vi "XMLExtractSheets.vi"(8 "error in (no error)":errorcluster, 11 "byte stream":string="<?xml version=\"1.0\" encoding=\"UTF-8\"?>\n<office:document-content xmlns:office=\"urn:oasis:names:tc:opendocument:xmlns:office:1.0\" xmlns:style=\"urn:oasis:names:tc:opendocument:xmlns:style:1.0\" xmlns:text=\"urn:oasis:names:tc:opendocument:xmlns:text:1.0\" xmlns:table=\"urn:oasis:names:tc:opendocument:xmlns:table:1.0\" xmlns:draw=\"urn:oasis:names:tc:opendocument:xmlns:drawing:1.0\" xmlns:fo=\"urn:oasis:names:tc:opendocument:xmlns:xsl-fo-compatible:1.0\" xmlns:xlink=\"http://www.w3.org/1999/xlink\" xmlns:dc=\"http://purl.org/dc/elements/1.1/\" xmlns:meta=\"urn:oasis:names:tc:opendocument:xmlns:meta:1.0\" xmlns:number=\"urn:oasis:names:tc:opendocument:xmlns:datastyle:1.0\" xmlns:presentation=\"urn:oasis:names:tc:opendocument:xmlns:presentation:1.0\" xmlns:svg=\"urn:oasis:names:tc:opendocument:xmlns:svg-compatible:1.0\" xmlns:chart=\"urn:oasis:names:tc:opendocument:xmlns:chart:1.0\" xmlns:dr3d=\"urn:oasis:names:tc:opendocument:xmlns:dr3d:1.0\" xmlns:math=\"http://www.w3.org/1998/Math/MathML\" xmlns:form=\"urn:oasis:names:tc:opendocument:xmlns:form:1.0\" xmlns:script=\"urn:oasis:names:tc:opendocument:xmlns:script:1.0\" xmlns:ooo=\"http://openoffice.org/2004/office\" xmlns:ooow=\"http://openoffice.org/2004/writer\" xmlns:oooc=\"http://openoffice.org/2004/calc\" xmlns:dom=\"http://www.w3.org/2001/xml-events\" xmlns:xforms=\"http://www.w3.org/2002/xforms\" xmlns:xsd=\"http://www.w3.org/2001/XMLSchema\" xmlns:xsi=\"http://www.w3.org/2001/XMLSchema-instance\" xmlns:rpt=\"http://openoffice.org/2005/report\" xmlns:of=\"urn:oasis:names:tc:opendocument:xmlns:of:1.2\" xmlns:xhtml=\"http://www.w3.org/1999/xhtml\" xmlns:grddl=\"http://www.w3.org/2003/g/data-view#\" xmlns:tableooo=\"http://openoffice.org/2009/table\" xmlns:drawooo=\"http://openoffice.org/2010/draw\" xmlns:calcext=\"urn:org:documentfoundation:names:experimental:calc:xmlns:calcext:1.0\" xmlns:loext=\"urn:org:documentfoundation:names:experimental:office:xmlns:loext:1.0\" xmlns:field=\"urn:openoffice:names:experimental:ooo-ms-interop:xmlns:field:1.0\" xmlns:formx=\"urn:openoffice:names:experimental:ooxml-odf-interop:xmlns:form:1.0\" xmlns:css3t=\"http://www.w3.org/TR/css3-text/\" office:version=\"1.2\"><office:scripts/><office:font-face-decls><style:font-face style:name=\"Liberation Sans\" svg:font-family=\"&apos;Liberation Sans&apos;\" style:font-family-generic=\"swiss\" style:font-pitch=\"variable\"/><style:font-face style:name=\"Mangal\" svg:font-family=\"Mangal\" style:font-family-generic=\"system\" style:font-pitch=\"variable\"/><style:font-face style:name=\"Microsoft YaHei\" svg:font-family=\"&apos;Microsoft YaHei&apos;\" style:font-family-generic=\"system\" style:font-pitch=\"variable\"/><style:font-face style:name=\"Segoe UI\" svg:font-family=\"&apos;Segoe UI&apos;\" style:font-family-generic=\"system\" style:font-pitch=\"variable\"/><style:font-face style:name=\"Tahoma\" svg:font-family=\"Tahoma\" style:font-family-generic=\"system\" style:font-pitch=\"variable\"/></office:font-face-decls><office:automatic-styles><style:style style:name=\"co1\" style:family=\"table-column\"><style:table-column-properties fo:break-before=\"auto\" style:column-width=\"22.58mm\"/></style:style><style:style style:name=\"ro1\" style:family=\"table-row\"><style:table-row-properties style:row-height=\"4.52mm\" fo:break-before=\"auto\" style:use-optimal-row-height=\"true\"/></style:style><style:style style:name=\"ta1\" style:family=\"table\" style:master-page-name=\"Default\"><style:table-properties table:display=\"true\" style:writing-mode=\"lr-tb\"/></style:style></office:automatic-styles><office:body><office:spreadsheet><table:table table:name=\"Sheet1\" table:style-name=\"ta1\"><table:table-column table:style-name=\"co1\" table:number-columns-repeated=\"8\" table:default-cell-style-name=\"Default\"/><table:table-row table:style-name=\"ro1\" table:number-rows-repeated=\"3\"><table:table-cell table:number-columns-repeated=\"8\"/></table:table-row><table:table-row table:style-name=\"ro1\"><table:table-cell/><table:table-cell office:value-type=\"string\" calcext:value-type=\"string\"><text:p>b1</text:p></table:table-cell><table:table-cell office:value-type=\"string\" calcext:value-type=\"string\"><text:p>c1</text:p></table:table-cell><table:table-cell table:number-columns-repeated=\"5\"/></table:table-row><table:table-row table:style-name=\"ro1\"><table:table-cell/><table:table-cell office:value-type=\"string\" calcext:value-type=\"string\"><text:p>b2</text:p></table:table-cell><table:table-cell office:value-type=\"string\" calcext:value-type=\"string\"><text:p>c2</text:p></table:table-cell><table:table-cell table:number-columns-repeated=\"5\"/></table:table-row><table:table-row table:style-name=\"ro1\"><table:table-cell/><table:table-cell office:value-type=\"string\" calcext:value-type=\"string\"><text:p>b3</text:p></table:table-cell><table:table-cell office:value-type=\"string\" calcext:value-type=\"string\"><text:p>c3</text:p></table:table-cell><table:table-cell table:number-columns-repeated=\"5\"/></table:table-row><table:table-row table:style-name=\"ro1\"><table:table-cell/><table:table-cell office:value-type=\"string\" calcext:value-type=\"string\"><text:p>b4</text:p></table:table-cell><table:table-cell office:value-type=\"string\" calcext:value-type=\"string\"><text:p>c4</text:p></table:table-cell><table:table-cell table:number-columns-repeated=\"5\"/></table:table-row><table:table-row table:style-name=\"ro1\"><table:table-cell/><table:table-cell office:value-type=\"string\" calcext:value-type=\"string\"><text:p>b5</text:p></table:table-cell><table:table-cell office:value-type=\"string\" calcext:value-type=\"string\"><text:p>c5</text:p></table:table-cell><table:table-cell table:number-columns-repeated=\"5\"/></table:table-row><table:table-row table:style-name=\"ro1\"><table:table-cell/><table:table-cell office:value-type=\"string\" calcext:value-type=\"string\"><text:p>b6</text:p></table:table-cell><table:table-cell office:value-type=\"string\" calcext:value-type=\"string\"><text:p>c6</text:p></table:table-cell><table:table-cell table:number-columns-repeated=\"5\"/></table:table-row><table:table-row table:style-name=\"ro1\"><table:table-cell/><table:table-cell office:value-type=\"string\" calcext:value-type=\"string\"><text:p>b7</text:p></table:table-cell><table:table-cell office:value-type=\"string\" calcext:value-type=\"string\"><text:p>c7</text:p></table:table-cell><table:table-cell table:number-columns-repeated=\"5\"/></table:table-row><table:table-row table:style-name=\"ro1\"><table:table-cell/><table:table-cell office:value-type=\"string\" calcext:value-type=\"string\"><text:p>b8</text:p></table:table-cell><table:table-cell office:value-type=\"string\" calcext:value-type=\"string\"><text:p>c8</text:p></table:table-cell><table:table-cell table:number-columns-repeated=\"5\"/></table:table-row><table:table-row table:style-name=\"ro1\" table:number-rows-repeated=\"2\"><table:table-cell table:number-columns-repeated=\"8\"/></table:table-row><table:table-row table:style-name=\"ro1\"><table:table-cell table:number-columns-repeated=\"3\"/><table:table-cell office:value-type=\"string\" calcext:value-type=\"string\"><text:p>d1</text:p></table:table-cell><table:table-cell office:value-type=\"string\" calcext:value-type=\"string\"><text:p>e1</text:p></table:table-cell><table:table-cell table:number-columns-repeated=\"3\"/></table:table-row><table:table-row table:style-name=\"ro1\"><table:table-cell table:number-columns-repeated=\"3\"/><table:table-cell office:value-type=\"string\" calcext:value-type=\"string\"><text:p>d2</text:p></table:table-cell><table:table-cell office:value-type=\"string\" calcext:value-type=\"string\"><text:p>e2</text:p></table:table-cell><table:table-cell table:number-columns-repeated=\"3\"/></table:table-row><table:table-row table:style-name=\"ro1\"><table:table-cell table:number-columns-repeated=\"3\"/><table:table-cell office:value-type=\"string\" calcext:value-type=\"string\"><text:p>d3</text:p></table:table-cell><table:table-cell office:value-type=\"string\" calcext:value-type=\"string\"><text:p>e3</text:p></table:table-cell><table:table-cell table:number-columns-repeated=\"3\"/></table:table-row><table:table-row table:style-name=\"ro1\"><table:table-cell table:number-columns-repeated=\"3\"/><table:table-cell office:value-type=\"string\" calcext:value-type=\"string\"><text:p>d4</text:p></table:table-cell><table:table-cell office:value-type=\"string\" calcext:value-type=\"string\"><text:p>e4</text:p></table:table-cell><table:table-cell table:number-columns-repeated=\"3\"/></table:table-row><table:table-row table:style-name=\"ro1\"><table:table-cell table:number-columns-repeated=\"3\"/><table:table-cell office:value-type=\"string\" calcext:value-type=\"string\"><text:p>d5</text:p></table:table-cell><table:table-cell office:value-type=\"string\" calcext:value-type=\"string\"><text:p>e5</text:p></table:table-cell><table:table-cell table:number-columns-repeated=\"3\"/></table:table-row><table:table-row table:style-name=\"ro1\" table:number-rows-repeated=\"14\"><table:table-cell table:number-columns-repeated=\"8\"/></table:table-row><table:table-row table:style-name=\"ro1\"><table:table-cell table:number-columns-repeated=\"5\"/><table:table-cell office:value-type=\"string\" calcext:value-type=\"string\"><text:p>f1</text:p></table:table-cell><table:table-cell/><table:table-cell office:value-type=\"string\" calcext:value-type=\"string\"><text:p>h1</text:p></table:table-cell></table:table-row><table:table-row table:style-name=\"ro1\"><table:table-cell table:number-columns-repeated=\"5\"/><table:table-cell office:value-type=\"string\" calcext:value-type=\"string\"><text:p>f2</text:p></table:table-cell><table:table-cell/><table:table-cell office:value-type=\"string\" calcext:value-type=\"string\"><text:p>h2</text:p></table:table-cell></table:table-row><table:table-row table:style-name=\"ro1\"><table:table-cell table:number-columns-repeated=\"5\"/><table:table-cell office:value-type=\"string\" calcext:value-type=\"string\"><text:p>f3</text:p></table:table-cell><table:table-cell/><table:table-cell office:value-type=\"string\" calcext:value-type=\"string\"><text:p>h3</text:p></table:table-cell></table:table-row><table:table-row table:style-name=\"ro1\"><table:table-cell table:number-columns-repeated=\"5\"/><table:table-cell office:value-type=\"string\" calcext:value-type=\"string\"><text:p>f4</text:p></table:table-cell><table:table-cell/><table:table-cell office:value-type=\"string\" calcext:value-type=\"string\"><text:p>h4</text:p></table:table-cell></table:table-row><table:table-row table:style-name=\"ro1\"><table:table-cell table:number-columns-repeated=\"5\"/><table:table-cell office:value-type=\"string\" calcext:value-type=\"string\"><text:p>f5</text:p></table:table-cell><table:table-cell/><table:table-cell office:value-type=\"string\" calcext:value-type=\"string\"><text:p>h5</text:p></table:table-cell></table:table-row><table:table-row table:style-name=\"ro1\"><table:table-cell table:number-columns-repeated=\"5\"/><table:table-cell office:value-type=\"string\" calcext:value-type=\"string\"><text:p>f6</text:p></table:table-cell><table:table-cell/><table:table-cell office:value-type=\"string\" calcext:value-type=\"string\"><text:p>h6</text:p></table:table-cell></table:table-row><table:table-row table:style-name=\"ro1\"><table:table-cell table:number-columns-repeated=\"5\"/><table:table-cell office:value-type=\"string\" calcext:value-type=\"string\"><text:p>f7</text:p></table:table-cell><table:table-cell/><table:table-cell office:value-type=\"string\" calcext:value-type=\"string\"><text:p>h7</text:p></table:table-cell></table:table-row></table:table><table:table table:name=\"Sheet1_2\" table:style-name=\"ta1\"><table:table-column table:style-name=\"co1\" table:number-columns-repeated=\"8\" table:default-cell-style-name=\"Default\"/><table:table-row table:style-name=\"ro1\" table:number-rows-repeated=\"3\"><table:table-cell table:number-columns-repeated=\"8\"/></table:table-row><table:table-row table:style-name=\"ro1\"><table:table-cell/><table:table-cell office:value-type=\"string\" calcext:value-type=\"string\"><text:p>b1</text:p></table:table-cell><table:table-cell office:value-type=\"string\" calcext:value-type=\"string\"><text:p>c1</text:p></table:table-cell><table:table-cell table:number-columns-repeated=\"5\"/></table:table-row><table:table-row table:style-name=\"ro1\"><table:table-cell/><table:table-cell office:value-type=\"string\" calcext:value-type=\"string\"><text:p>b2</text:p></table:table-cell><table:table-cell office:value-type=\"string\" calcext:value-type=\"string\"><text:p>c2</text:p></table:table-cell><table:table-cell table:number-columns-repeated=\"5\"/></table:table-row><table:table-row table:style-name=\"ro1\"><table:table-cell/><table:table-cell office:value-type=\"string\" calcext:value-type=\"string\"><text:p>b3</text:p></table:table-cell><table:table-cell office:value-type=\"string\" calcext:value-type=\"string\"><text:p>c3</text:p></table:table-cell><table:table-cell table:number-columns-repeated=\"5\"/></table:table-row><table:table-row table:style-name=\"ro1\"><table:table-cell/><table:table-cell office:value-type=\"string\" calcext:value-type=\"string\"><text:p>b4</text:p></table:table-cell><table:table-cell office:value-type=\"string\" calcext:value-type=\"string\"><text:p>c4</text:p></table:table-cell><table:table-cell table:number-columns-repeated=\"5\"/></table:table-row><table:table-row table:style-name=\"ro1\"><table:table-cell/><table:table-cell office:value-type=\"string\" calcext:value-type=\"string\"><text:p>b5</text:p></table:table-cell><table:table-cell office:value-type=\"string\" calcext:value-type=\"string\"><text:p>c5</text:p></table:table-cell><table:table-cell table:number-columns-repeated=\"5\"/></table:table-row><table:table-row table:style-name=\"ro1\"><table:table-cell/><table:table-cell office:value-type=\"string\" calcext:value-type=\"string\"><text:p>b6</text:p></table:table-cell><table:table-cell office:value-type=\"string\" calcext:value-type=\"string\"><text:p>c6</text:p></table:table-cell><table:table-cell table:number-columns-repeated=\"5\"/></table:table-row><table:table-row table:style-name=\"ro1\"><table:table-cell/><table:table-cell office:value-type=\"string\" calcext:value-type=\"string\"><text:p>b7</text:p></table:table-cell><table:table-cell office:value-type=\"string\" calcext:value-type=\"string\"><text:p>c7</text:p></table:table-cell><table:table-cell table:number-columns-repeated=\"5\"/></table:table-row><table:table-row table:style-name=\"ro1\"><table:table-cell/><table:table-cell office:value-type=\"string\" calcext:value-type=\"string\"><text:p>b8</text:p></table:table-cell><table:table-cell office:value-type=\"string\" calcext:value-type=\"string\"><text:p>c8</text:p></table:table-cell><table:table-cell table:number-columns-repeated=\"5\"/></table:table-row><table:table-row table:style-name=\"ro1\" table:number-rows-repeated=\"2\"><table:table-cell table:number-columns-repeated=\"8\"/></table:table-row><table:table-row table:style-name=\"ro1\"><table:table-cell table:number-columns-repeated=\"3\"/><table:table-cell office:value-type=\"string\" calcext:value-type=\"string\"><text:p>d1</text:p></table:table-cell><table:table-cell office:value-type=\"string\" calcext:value-type=\"string\"><text:p>e1</text:p></table:table-cell><table:table-cell table:number-columns-repeated=\"3\"/></table:table-row><table:table-row table:style-name=\"ro1\"><table:table-cell table:number-columns-repeated=\"3\"/><table:table-cell office:value-type=\"string\" calcext:value-type=\"string\"><text:p>d2</text:p></table:table-cell><table:table-cell office:value-type=\"string\" calcext:value-type=\"string\"><text:p>e2</text:p></table:table-cell><table:table-cell table:number-columns-repeated=\"3\"/></table:table-row><table:table-row table:style-name=\"ro1\"><table:table-cell table:number-columns-repeated=\"3\"/><table:table-cell office:value-type=\"string\" calcext:value-type=\"string\"><text:p>d3</text:p></table:table-cell><table:table-cell office:value-type=\"string\" calcext:value-type=\"string\"><text:p>e3</text:p></table:table-cell><table:table-cell table:number-columns-repeated=\"3\"/></table:table-row><table:table-row table:style-name=\"ro1\"><table:table-cell table:number-columns-repeated=\"3\"/><table:table-cell office:value-type=\"string\" calcext:value-type=\"string\"><text:p>d4</text:p></table:table-cell><table:table-cell office:value-type=\"string\" calcext:value-type=\"string\"><text:p>e4</text:p></table:table-cell><table:table-cell table:number-columns-repeated=\"3\"/></table:table-row><table:table-row table:style-name=\"ro1\"><table:table-cell table:number-columns-repeated=\"3\"/><table:table-cell office:value-type=\"string\" calcext:value-type=\"string\"><text:p>d5</text:p></table:table-cell><table:table-cell office:value-type=\"string\" calcext:value-type=\"string\"><text:p>e5</text:p></table:table-cell><table:table-cell table:number-columns-repeated=\"3\"/></table:table-row><table:table-row table:style-name=\"ro1\" table:number-rows-repeated=\"14\"><table:table-cell table:number-columns-repeated=\"8\"/></table:table-row><table:table-row table:style-name=\"ro1\"><table:table-cell/><table:table-cell office:value-type=\"string\" calcext:value-type=\"string\"><text:p>f1</text:p></table:table-cell><table:table-cell table:number-columns-repeated=\"5\"/><table:table-cell office:value-type=\"string\" calcext:value-type=\"string\"><text:p>h1</text:p></table:table-cell></table:table-row><table:table-row table:style-name=\"ro1\"><table:table-cell/><table:table-cell office:value-type=\"string\" calcext:value-type=\"string\"><text:p>f2</text:p></table:table-cell><table:table-cell table:number-columns-repeated=\"5\"/><table:table-cell office:value-type=\"string\" calcext:value-type=\"string\"><text:p>h2</text:p></table:table-cell></table:table-row><table:table-row table:style-name=\"ro1\"><table:table-cell/><table:table-cell office:value-type=\"string\" calcext:value-type=\"string\"><text:p>f3</text:p></table:table-cell><table:table-cell table:number-columns-repeated=\"5\"/><table:table-cell office:value-type=\"string\" calcext:value-type=\"string\"><text:p>h3</text:p></table:table-cell></table:table-row><table:table-row table:style-name=\"ro1\"><table:table-cell/><table:table-cell office:value-type=\"string\" calcext:value-type=\"string\"><text:p>f4</text:p></table:table-cell><table:table-cell table:number-columns-repeated=\"5\"/><table:table-cell office:value-type=\"string\" calcext:value-type=\"string\"><text:p>h4</text:p></table:table-cell></table:table-row><table:table-row table:style-name=\"ro1\"><table:table-cell/><table:table-cell office:value-type=\"string\" calcext:value-type=\"string\"><text:p>f5</text:p></table:table-cell><table:table-cell table:number-columns-repeated=\"5\"/><table:table-cell office:value-type=\"string\" calcext:value-type=\"string\"><text:p>h5</text:p></table:table-cell></table:table-row><table:table-row table:style-name=\"ro1\"><table:table-cell/><table:table-cell office:value-type=\"string\" calcext:value-type=\"string\"><text:p>f6</text:p></table:table-cell><table:table-cell table:number-columns-repeated=\"5\"/><table:table-cell office:value-type=\"string\" calcext:value-type=\"string\"><text:p>h6</text:p></table:table-cell></table:table-row><table:table-row table:style-name=\"ro1\"><table:table-cell/><table:table-cell office:value-type=\"string\" calcext:value-type=\"string\"><text:p>f7</text:p></table:table-cell><table:table-cell table:number-columns-repeated=\"5\"/><table:table-cell office:value-type=\"string\" calcext:value-type=\"string\"><text:p>h7</text:p></table:table-cell></table:table-row></table:table><table:named-expressions/></office:spreadsheet></office:body></office:document-content>") -> (0 "error out":errorcluster, 1 "Footer":string="</office:body></office:document-content>", 2 "Sheets":string[](array[string])=["<table:table table:name=\"Sheet1\" table:style-name=\"ta1\"><table:table-column table:style-name=\"co1\" table:number-columns-repeated=\"8\" table:default-cell-style-name=\"Default\"/><table:table-row table:style-name=\"ro1\" table:number-rows-repeated=\"3\"><table:table-cell table:number-columns-repeated=\"8\"/></table:table-row><table:table-row table:style-name=\"ro1\"><table:table-cell/><table:table-cell office:value-type=\"string\" calcext:value-type=\"string\"><text:p>b1</text:p></table:table-cell><table:table-cell office:value-type=\"string\" calcext:value-type=\"string\"><text:p>c1</text:p></table:table-cell><table:table-cell table:number-columns-repeated=\"5\"/></table:table-row><table:table-row table:style-name=\"ro1\"><table:table-cell/><table:table-cell office:value-type=\"string\" calcext:value-type=\"string\"><text:p>b2</text:p></table:table-cell><table:table-cell office:value-type=\"string\" calcext:value-type=\"string\"><text:p>c2</text:p></table:table-cell><table:table-cell table:number-columns-repeated=\"5\"/></table:table-row><table:table-row table:style-name=\"ro1\"><table:table-cell/><table:table-cell office:value-type=\"string\" calcext:value-type=\"string\"><text:p>b3</text:p></table:table-cell><table:table-cell office:value-type=\"string\" calcext:value-type=\"string\"><text:p>c3</text:p></table:table-cell><table:table-cell table:number-columns-repeated=\"5\"/></table:table-row><table:table-row table:style-name=\"ro1\"><table:table-cell/><table:table-cell office:value-type=\"string\" calcext:value-type=\"string\"><text:p>b4</text:p></table:table-cell><table:table-cell office:value-type=\"string\" calcext:value-type=\"string\"><text:p>c4</text:p></table:table-cell><table:table-cell table:number-columns-repeated=\"5\"/></table:table-row><table:table-row table:style-name=\"ro1\"><table:table-cell/><table:table-cell office:value-type=\"string\" calcext:value-type=\"string\"><text:p>b5</text:p></table:table-cell><table:table-cell office:value-type=\"string\" calcext:value-type=\"string\"><text:p>c5</text:p></table:table-cell><table:table-cell table:number-columns-repeated=\"5\"/></table:table-row><table:table-row table:style-name=\"ro1\"><table:table-cell/><table:table-cell office:value-type=\"string\" calcext:value-type=\"string\"><text:p>b6</text:p></table:table-cell><table:table-cell office:value-type=\"string\" calcext:value-type=\"string\"><text:p>c6</text:p></table:table-cell><table:table-cell table:number-columns-repeated=\"5\"/></table:table-row><table:table-row table:style-name=\"ro1\"><table:table-cell/><table:table-cell office:value-type=\"string\" calcext:value-type=\"string\"><text:p>b7</text:p></table:table-cell><table:table-cell office:value-type=\"string\" calcext:value-type=\"string\"><text:p>c7</text:p></table:table-cell><table:table-cell table:number-columns-repeated=\"5\"/></table:table-row><table:table-row table:style-name=\"ro1\"><table:table-cell/><table:table-cell office:value-type=\"string\" calcext:value-type=\"string\"><text:p>b8</text:p></table:table-cell><table:table-cell office:value-type=\"string\" calcext:value-type=\"string\"><text:p>c8</text:p></table:table-cell><table:table-cell table:number-columns-repeated=\"5\"/></table:table-row><table:table-row table:style-name=\"ro1\" table:number-rows-repeated=\"2\"><table:table-cell table:number-columns-repeated=\"8\"/></table:table-row><table:table-row table:style-name=\"ro1\"><table:table-cell table:number-columns-repeated=\"3\"/><table:table-cell office:value-type=\"string\" calcext:value-type=\"string\"><text:p>d1</text:p></table:table-cell><table:table-cell office:value-type=\"string\" calcext:value-type=\"string\"><text:p>e1</text:p></table:table-cell><table:table-cell table:number-columns-repeated=\"3\"/></table:table-row><table:table-row table:style-name=\"ro1\"><table:table-cell table:number-columns-repeated=\"3\"/><table:table-cell office:value-type=\"string\" calcext:value-type=\"string\"><text:p>d2</text:p></table:table-cell><table:table-cell office:value-type=\"string\" calcext:value-type=\"string\"><text:p>e2</text:p></table:table-cell><table:table-cell table:number-columns-repeated=\"3\"/></table:table-row><table:table-row table:style-name=\"ro1\"><table:table-cell table:number-columns-repeated=\"3\"/><table:table-cell office:value-type=\"string\" calcext:value-type=\"string\"><text:p>d3</text:p></table:table-cell><table:table-cell office:value-type=\"string\" calcext:value-type=\"string\"><text:p>e3</text:p></table:table-cell><table:table-cell table:number-columns-repeated=\"3\"/></table:table-row><table:table-row table:style-name=\"ro1\"><table:table-cell table:number-columns-repeated=\"3\"/><table:table-cell office:value-type=\"string\" calcext:value-type=\"string\"><text:p>d4</text:p></table:table-cell><table:table-cell office:value-type=\"string\" calcext:value-type=\"string\"><text:p>e4</text:p></table:table-cell><table:table-cell table:number-columns-repeated=\"3\"/></table:table-row><table:table-row table:style-name=\"ro1\"><table:table-cell table:number-columns-repeated=\"3\"/><table:table-cell office:value-type=\"string\" calcext:value-type=\"string\"><text:p>d5</text:p></table:table-cell><table:table-cell office:value-type=\"string\" calcext:value-type=\"string\"><text:p>e5</text:p></table:table-cell><table:table-cell table:number-columns-repeated=\"3\"/></table:table-row><table:table-row table:style-name=\"ro1\" table:number-rows-repeated=\"14\"><table:table-cell table:number-columns-repeated=\"8\"/></table:table-row><table:table-row table:style-name=\"ro1\"><table:table-cell table:number-columns-repeated=\"5\"/><table:table-cell office:value-type=\"string\" calcext:value-type=\"string\"><text:p>f1</text:p></table:table-cell><table:table-cell/><table:table-cell office:value-type=\"string\" calcext:value-type=\"string\"><text:p>h1</text:p></table:table-cell></table:table-row><table:table-row table:style-name=\"ro1\"><table:table-cell table:number-columns-repeated=\"5\"/><table:table-cell office:value-type=\"string\" calcext:value-type=\"string\"><text:p>f2</text:p></table:table-cell><table:table-cell/><table:table-cell office:value-type=\"string\" calcext:value-type=\"string\"><text:p>h2</text:p></table:table-cell></table:table-row><table:table-row table:style-name=\"ro1\"><table:table-cell table:number-columns-repeated=\"5\"/><table:table-cell office:value-type=\"string\" calcext:value-type=\"string\"><text:p>f3</text:p></table:table-cell><table:table-cell/><table:table-cell office:value-type=\"string\" calcext:value-type=\"string\"><text:p>h3</text:p></table:table-cell></table:table-row><table:table-row table:style-name=\"ro1\"><table:table-cell table:number-columns-repeated=\"5\"/><table:table-cell office:value-type=\"string\" calcext:value-type=\"string\"><text:p>f4</text:p></table:table-cell><table:table-cell/><table:table-cell office:value-type=\"string\" calcext:value-type=\"string\"><text:p>h4</text:p></table:table-cell></table:table-row><table:table-row table:style-name=\"ro1\"><table:table-cell table:number-columns-repeated=\"5\"/><table:table-cell office:value-type=\"string\" calcext:value-type=\"string\"><text:p>f5</text:p></table:table-cell><table:table-cell/><table:table-cell office:value-type=\"string\" calcext:value-type=\"string\"><text:p>h5</text:p></table:table-cell></table:table-row><table:table-row table:style-name=\"ro1\"><table:table-cell table:number-columns-repeated=\"5\"/><table:table-cell office:value-type=\"string\" calcext:value-type=\"string\"><text:p>f6</text:p></table:table-cell><table:table-cell/><table:table-cell office:value-type=\"string\" calcext:value-type=\"string\"><text:p>h6</text:p></table:table-cell></table:table-row><table:table-row table:style-name=\"ro1\"><table:table-cell table:number-columns-repeated=\"5\"/><table:table-cell office:value-type=\"string\" calcext:value-type=\"string\"><text:p>f7</text:p></table:table-cell><table:table-cell/><table:table-cell office:value-type=\"string\" calcext:value-type=\"string\"><text:p>h7</text:p></table:table-cell></table:table-row></table:table>"], 3 "Header":string="<?xml version=\"1.0\" encoding=\"UTF-8\"?>\n<office:document-content xmlns:office=\"urn:oasis:names:tc:opendocument:xmlns:office:1.0\" xmlns:style=\"urn:oasis:names:tc:opendocument:xmlns:style:1.0\" xmlns:text=\"urn:oasis:names:tc:opendocument:xmlns:text:1.0\" xmlns:table=\"urn:oasis:names:tc:opendocument:xmlns:table:1.0\" xmlns:draw=\"urn:oasis:names:tc:opendocument:xmlns:drawing:1.0\" xmlns:fo=\"urn:oasis:names:tc:opendocument:xmlns:xsl-fo-compatible:1.0\" xmlns:xlink=\"http://www.w3.org/1999/xlink\" xmlns:dc=\"http://purl.org/dc/elements/1.1/\" xmlns:meta=\"urn:oasis:names:tc:opendocument:xmlns:meta:1.0\" xmlns:number=\"urn:oasis:names:tc:opendocument:xmlns:datastyle:1.0\" xmlns:presentation=\"urn:oasis:names:tc:opendocument:xmlns:presentation:1.0\" xmlns:svg=\"urn:oasis:names:tc:opendocument:xmlns:svg-compatible:1.0\" xmlns:chart=\"urn:oasis:names:tc:opendocument:xmlns:chart:1.0\" xmlns:dr3d=\"urn:oasis:names:tc:opendocument:xmlns:dr3d:1.0\" xmlns:math=\"http://www.w3.org/1998/Math/MathML\" xmlns:form=\"urn:oasis:names:tc:opendocument:xmlns:form:1.0\" xmlns:script=\"urn:oasis:names:tc:opendocument:xmlns:script:1.0\" xmlns:ooo=\"http://openoffice.org/2004/office\" xmlns:ooow=\"http://openoffice.org/2004/writer\" xmlns:oooc=\"http://openoffice.org/2004/calc\" xmlns:dom=\"http://www.w3.org/2001/xml-events\" xmlns:xforms=\"http://www.w3.org/2002/xforms\" xmlns:xsd=\"http://www.w3.org/2001/XMLSchema\" xmlns:xsi=\"http://www.w3.org/2001/XMLSchema-instance\" xmlns:rpt=\"http://openoffice.org/2005/report\" xmlns:of=\"urn:oasis:names:tc:opendocument:xmlns:of:1.2\" xmlns:xhtml=\"http://www.w3.org/1999/xhtml\" xmlns:grddl=\"http://www.w3.org/2003/g/data-view#\" xmlns:tableooo=\"http://openoffice.org/2009/table\" xmlns:drawooo=\"http://openoffice.org/2010/draw\" xmlns:calcext=\"urn:org:documentfoundation:names:experimental:calc:xmlns:calcext:1.0\" xmlns:loext=\"urn:org:documentfoundation:names:experimental:office:xmlns:loext:1.0\" xmlns:field=\"urn:openoffice:names:experimental:ooo-ms-interop:xmlns:field:1.0\" xmlns:formx=\"urn:openoffice:names:experimental:ooxml-odf-interop:xmlns:form:1.0\" xmlns:css3t=\"http://www.w3.org/TR/css3-text/\" office:version=\"1.2\"><office:scripts/><office:font-face-decls><style:font-face style:name=\"Liberation Sans\" svg:font-family=\"&apos;Liberation Sans&apos;\" style:font-family-generic=\"swiss\" style:font-pitch=\"variable\"/><style:font-face style:name=\"Mangal\" svg:font-family=\"Mangal\" style:font-family-generic=\"system\" style:font-pitch=\"variable\"/><style:font-face style:name=\"Microsoft YaHei\" svg:font-family=\"&apos;Microsoft YaHei&apos;\" style:font-family-generic=\"system\" style:font-pitch=\"variable\"/><style:font-face style:name=\"Segoe UI\" svg:font-family=\"&apos;Segoe UI&apos;\" style:font-family-generic=\"system\" style:font-pitch=\"variable\"/><style:font-face style:name=\"Tahoma\" svg:font-family=\"Tahoma\" style:font-family-generic=\"system\" style:font-pitch=\"variable\"/></office:font-face-decls><office:automatic-styles><style:style style:name=\"co1\" style:family=\"table-column\"><style:table-column-properties fo:break-before=\"auto\" style:column-width=\"22.58mm\"/></style:style><style:style style:name=\"ro1\" style:family=\"table-row\"><style:table-row-properties style:row-height=\"4.52mm\" fo:break-before=\"auto\" style:use-optimal-row-height=\"true\"/></style:style><style:style style:name=\"ta1\" style:family=\"table\" style:master-page-name=\"Default\"><style:table-properties table:display=\"true\" style:writing-mode=\"lr-tb\"/></style:style></office:automatic-styles><office:body>")   [LabVIEW 2014]
uses:
  <vilib>/regexp/Match Regular Expression.xnode
panel:
  # "Output"
  # "Input"
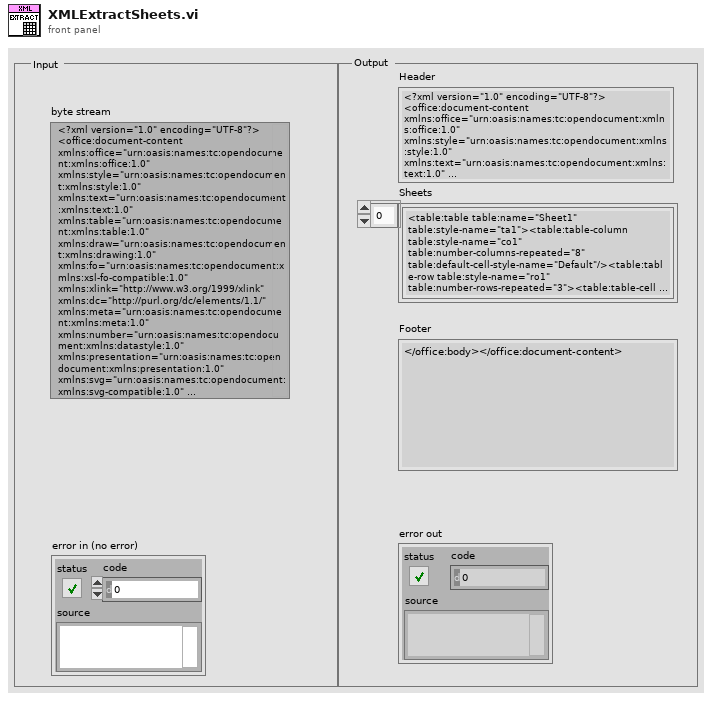
[diagram p1: front panel]
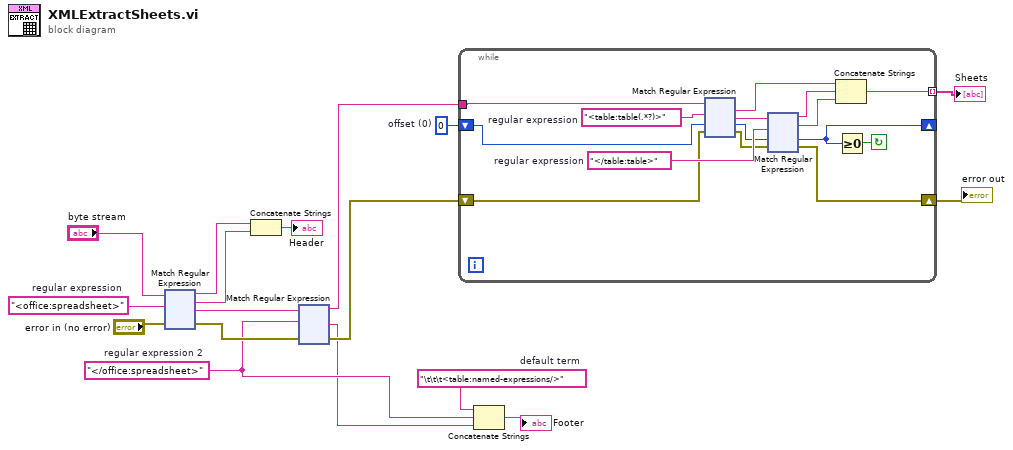
[diagram p0: block diagram]
diagram:
  w1 = "\t\t\t<table:named-expressions/>"  # default term
  w6 = "</office:spreadsheet>"  # regular expression 2
  w15 = "<office:spreadsheet>"  # regular expression
  w12 = 0  # offset (0)
  n1 = xnode "Match Regular Expression"("input string"="byte stream", "regular expression"=w15, "error in"="error in (no error)") -> ("before match"=w4:string, "whole match"=w3:string, "after match"=w14:string, "error out"=w13:errorcluster)  [unwired: 3 in, 1 out]
  n2 = Concatenate Strings(w4, w3) -> (→"Header":string)
  n3 = xnode "Match Regular Expression"("input string"=w14, "regular expression"=w6, "error in"=w13) -> ("before match"=w11:string, "after match"=w5:string, "error out"=w9:errorcluster)  [unwired: 3 in, 2 out]
  n4 = while {
    shift-right: [w22] -> _
    shift-left: w12 -> [w28]
    tunnel: w11 -> [w29]
    tunnel: [w23] -> w10 mode=indexing
    shift-right: [w20] -> w8
    shift-left: w9 -> [w19]
    stop <- w21 continue-if-true
    w30 = "</table:table>"  # regular expression
    w32 = "<table:table(.*?)>"  # regular expression
    n5 = xnode "Match Regular Expression"("input string"=w29, "regular expression"=w32, "offset (0)"=w28, "error in"=w19) -> ("whole match"=w24:string, "after match"=w31:string, "offset past match"=w27:i32, "error out"=w18:errorcluster)  [unwired: 2 in, 1 out]
    n6 = xnode "Match Regular Expression"("input string"=w31, "regular expression"=w30, "offset (0)"=w27, "error in"=w18) -> ("before match"=w25:string, "whole match"=w26:string, "offset past match"=w22:i32, "error out"=w20:errorcluster)  [unwired: 2 in, 1 out]
    n7 = Concatenate Strings(w24, w25, w26) -> (w23:string)
    n8 = Greater Or Equal To 0?(x=w22) -> (x >= 0?=w21:bool)
  }
  "error out" <- w8
  "Sheets" <- w10
  n9 = Concatenate Strings(w1, w6, w5) -> (→"Footer":string)
